vi "Deinterleave AO Channels.vi"(7 "clear":bool, 10 "data valid":bool, 11 "interleaved data":i16[](array[numeric])=[0, 0, 0, 0, 0, 0, 0, 0, 0, 0, 0, 0, 0, 0, 0, 0, 0, 0, 0, 0, 0, 0, 0, 0, 0, 0, 0, 0, 0, 0, 0, 0]) -> (3 "channel array":cluster{fxp<+/-,12,1>[]}[](array[cluster]))   [LabVIEW 2021]
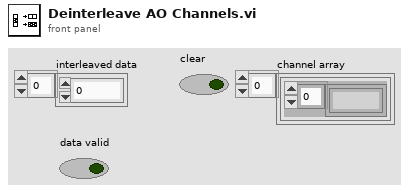
[diagram p1: front panel]
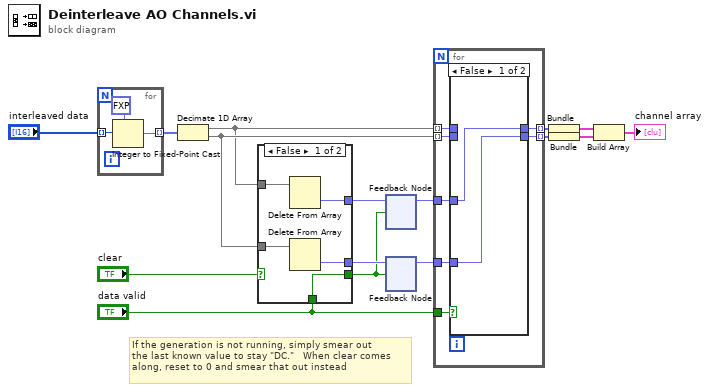
[diagram p0: block diagram]
diagram:
  # "If the generation is not running, simply smear out\nthe last known value to stay \"DC.\"   When clear comes along, reset to 0 and smear that out instead"
  n1 = for {
    tunnel: "interleaved data" -> [w19] mode=indexing
    tunnel: [w18] -> w13 mode=indexing
    n2 = Integer to Fixed-Point Cast(fixed-point type=fxp<+/-,12,1> 0.0 ("element"), integer=w19) -> (fixed-point=w18:fxp<+/-,12,1>)
  }
  n3 = Decimate 1D Array(w13) -> (w8:fxp<+/-,12,1>[], w9:fxp<+/-,12,1>[])
  n4 = case shown="False" "clear" {
    selector: "clear" -> [_ w25]
    tunnel: [w24 _] -> w11
    tunnel: [w23 _] -> w10
    tunnel: w9 -> [w22 _]
    tunnel: w8 -> [w21 _]
    tunnel: [w20 w25] -> w1
    tunnel: "data valid" -> [w20 _]
    frame False {
      n5 = Delete From Array(array=w21) -> (deleted portion=w24:fxp<+/-,12,1>)  [unwired: 2 in, 1 out]
      n6 = Delete From Array(array=w22) -> (deleted portion=w23:fxp<+/-,12,1>)  [unwired: 2 in, 1 out]
    }
    frame True {
    }
  }
  n7 = feedback-in #1(w11, w1) -> ()
  n8 = feedback #1() -> (w5:fxp<+/-,12,1>)  [unwired: 1 in]
  n9 = feedback #2() -> (w4:fxp<+/-,12,1>)  [unwired: 1 in]
  n10 = feedback-in #2(w10, w1) -> ()
  n11 = for {
    tunnel: w9 -> [w30] mode=indexing
    tunnel: w8 -> [w32] mode=indexing
    tunnel: [w31] -> w7 mode=indexing
    tunnel: [w29] -> w6 mode=indexing
    tunnel: "data valid" -> [w28]
    tunnel: w5 -> [w27]
    tunnel: w4 -> [w26]
    n12 = case shown="False" w28 {
      tunnel: [w34 w36] -> w31
      tunnel: w32 -> [_ w36]
      tunnel: w30 -> [_ w35]
      tunnel: [w33 w35] -> w29
      tunnel: w27 -> [w34 _]
      tunnel: w26 -> [w33 _]
      frame False {
      }
      frame True {
      }
    }
  }
  n13 = Bundle(w7) -> (w14:cluster{fxp<+/-,12,1>[]})  [unwired: 1 in]
  n14 = Bundle(w6) -> (w15:cluster{fxp<+/-,12,1>[]})  [unwired: 1 in]
  n15 = Build Array(w14, w15) -> (→"channel array":cluster{fxp<+/-,12,1>[]}[])
